vi "读输出状态.vi"(8 "error in (no error)":errorcluster, 11 "MB session in":refnum<class "MB_Master.lvclass">) -> (0 "error out":errorcluster, 2 "Coils":bool[](array[boolean]), 3 "MB session out":refnum<class "MB_Master.lvclass">)   [LabVIEW 2016, in "DAM395CF.lvlib"]
uses:
  DAM395CF.lvlib
  <vilib>/Plasmionique/MB Master/MB_Master/MB_Master.lvclass
  <vilib>/Plasmionique/MB Master/MB Master.lvlib
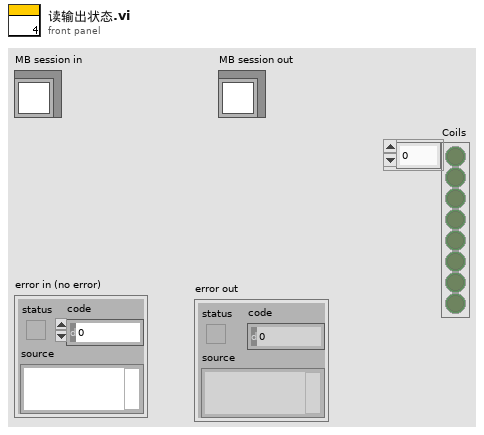
[diagram p1: front panel]
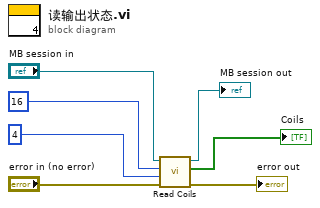
[diagram p0: block diagram]
diagram:
  n1 = call <vilib>:"Read Coils.vi"("error in (no error)"="error in (no error)", "quantity"=u16 4, "starting address"=u16 16, "MB session in"="MB session in") -> ("error out"=→"error out":errorcluster, "Coils"=→"Coils":bool[], "MB session out"=→"MB session out":refnum<class "MB_Master.lvclass">)  [unwired: 5 in]
